vi "Parse Variant.vi"(8 "error in":errorcluster, 10 "variant":variant) -> (0 "error out":errorcluster, 1 "Types":T1[](array[typedef]), 2 "Strings":string[](array[string]), 3 "Variants":variant[](array[variant]), 4 "Types (strings)":string[](array[string]))   [LabVIEW 2020, in "Data.PG.lvclass"]
uses:
  Data.PG.lvclass
  <vilib>/Utility/Data Type/NI_Data Type.lvlib
  <vilib>/Utility/Data Type/Type Definitions/Data Type.ctl
  <vilib>/ErrorRing/Error Ring.xnode
  <vilib>/Utility/error.llb/Error Cluster From Error Code.vi
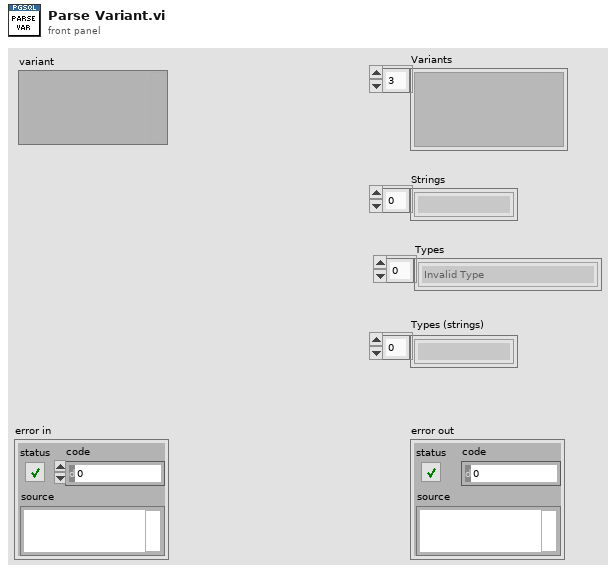
[diagram p1: front panel]
types:
  T1 = typedef "NI_Data Type.lvlib/Data Type.ctl" = enum8{"Invalid Type", "Void", "I8", "I16", "I32", "I64", "U8", "U16", "U32", "U64", "Single Float", "Double Float", "Extended Float", "Single Complex", "Double Complex", "Extended Complex", "Enum U8", "Enum U16", "Enum U32", "Enum U64", "Single Float With Unit", "Double Float With Unit", "Extended Float With Unit", "Single Complex with Unit", "Double Complex with Unit", "Extended Complex with Unit", "Boolean", "String", "Path", "Picture", "Tag", "Array", "Cluster", "Variant", "LV Variant", "Waveform", "Timestamp", "Digital Waveform", "Digital Data", "ExpressData", "Refnum", "External Data", "VI", "Poly VI", "LabVIEW Class Instance", "Fixed Point", "Set Collection", "Map Collection"}
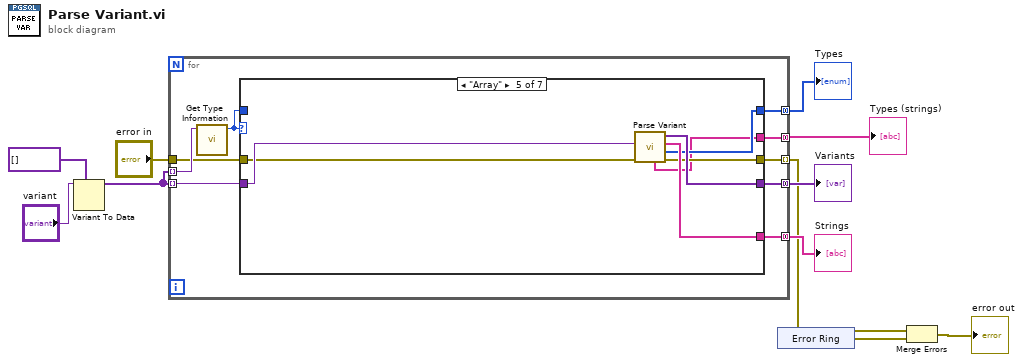
[diagram p0: block diagram]
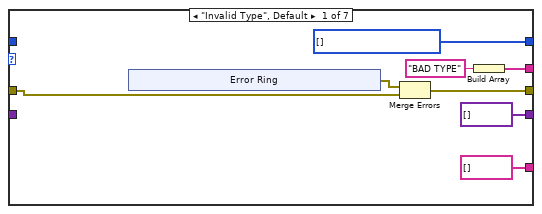
[diagram p2: hidden frame]
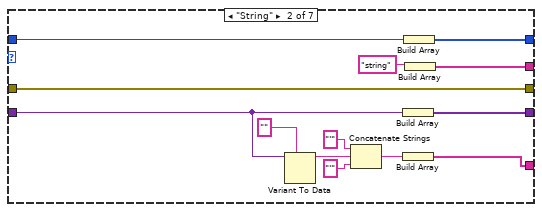
[diagram p3: hidden frame]
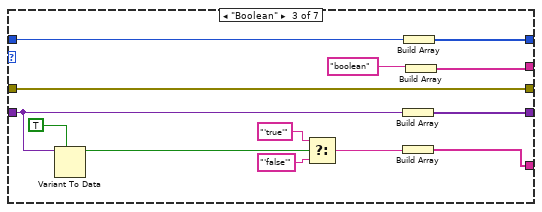
[diagram p4: hidden frame]
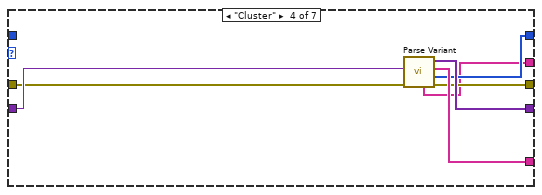
[diagram p5: hidden frame]
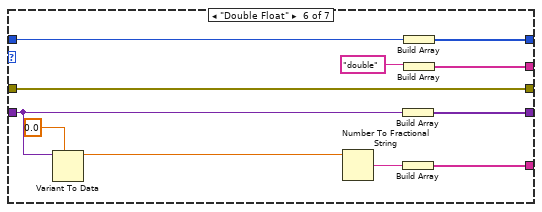
[diagram p6: hidden frame]
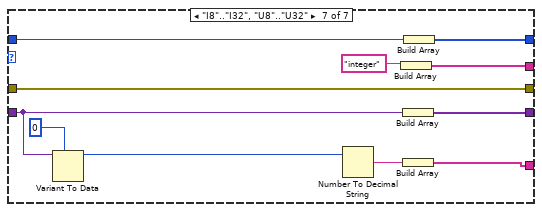
[diagram p7: hidden frame]
diagram:
  n1 = Variant To Data(type=variant[] [], Variant="variant") -> (data=w11:variant[])  [unwired: 1 in, 1 out]
  n2 = for {
    tunnel: w11 -> [w20] mode=indexing
    tunnel: w11 -> [w19] mode=indexing
    tunnel: [w17] -> w8 mode=concatenating
    tunnel: [w16] -> w7 mode=concatenating
    tunnel: [w15] -> w6 mode=concatenating
    tunnel: [w14] -> w4 mode=indexing
    tunnel: "error in" -> [w13]
    tunnel: [w12] -> w1 mode=concatenating
    n3 = call <vilib>:"Get Type Information.vi"("variant"=w20) -> ("type"=w18:T1)  [unwired: 6 in, 4 out]
    n4 = case shown="\"Array\"" w18 {
      tunnel: w19 -> [_ w38 w51 w66 w73 w77 w91]
      tunnel: [string[] [] ("Strings") w41 w54 w64 w71 w80 w89] -> w16
      tunnel: w18 -> [_ w39 w52 _ _ w82 w93]
      tunnel: [w26 w40 w53 w63 w70 w81 w92] -> w17
      tunnel: [variant[] [] ("Variants") w37 w50 w65 w72 w78 w90] -> w15
      tunnel: [w25 w36 w49 w62 w68 w76 w87] -> w14
      tunnel: w13 -> [w24 w36 w49 w61 w69 w76 w87]
      tunnel: [w22 w34 w47 w60 w67 w74 w85] -> w12
      frame "Invalid Type", Default {
        w26 = T1[] [] items=["Invalid Type", "Void", "I8", "I16", "I32", "I64", "U8", "U16", "U32", "U64", "Single Float", "Double Float", "Extended Float", "Single Complex", "Double Complex", "Extended Complex", "Enum U8", "Enum U16", "Enum U32", "Enum U64", "Single Float With Unit", "Double Float With Unit", "Extended Float With Unit", "Single Complex with Unit", "Double Complex with Unit", "Extended Complex with Unit", "Boolean", "String", "Path", "Picture", "Tag", "Array", "Cluster", "Variant", "LV Variant", "Waveform", "Timestamp", "Digital Waveform", "Digital Data", "ExpressData", "Refnum", "External Data", "VI", "Poly VI", "LabVIEW Class Instance", "Fixed Point", "Set Collection", "Map Collection"] ("Types")
        n5 = xnode "Error Ring"() -> ("error out"=w23:errorcluster)
        n6 = Merge Errors(w23, w24) -> (w25:errorcluster)
        n7 = Build Array("BAD TYPE") -> (w22:string[])
      }
      frame "String" {
        n8 = Variant To Data(type="", Variant=w38) -> (data=w45:string)  [unwired: 1 in, 1 out]
        n9 = Concatenate Strings("'" ("string"), w45, "'" ("string")) -> (w42:string)
        n10 = Build Array(w38) -> (w37:variant[])
        n11 = Build Array(w42) -> (w41:string[])
        n12 = Build Array(w39) -> (w40:T1[])
        n13 = Build Array("string") -> (w34:string[])
      }
      frame "Boolean" {
        n14 = Variant To Data(type=TRUE, Variant=w51) -> (data=w58:bool)  [unwired: 1 in, 1 out]
        n15 = Select(t="'true'", s=w58, f="'false'") -> (s? t:f=w55:string)
        n16 = Build Array(w51) -> (w50:variant[])
        n17 = Build Array(w55) -> (w54:string[])
        n18 = Build Array(w52) -> (w53:T1[])
        n19 = Build Array("boolean") -> (w47:string[])
      }
      frame "Cluster" {
        n20 = call "Parse Variant.vi"("error in"=w61, "variant"=w66) -> ("error out"=w62:errorcluster, "Types"=w63:T1[], "Strings"=w64:string[], "Variants"=w65:variant[], "Types (strings)"=w60:string[])  [unwired: 5 in]
      }
      frame "Array" {
        n21 = call "Parse Variant.vi"("error in"=w69, "variant"=w73) -> ("error out"=w68:errorcluster, "Types"=w70:T1[], "Strings"=w71:string[], "Variants"=w72:variant[], "Types (strings)"=w67:string[])  [unwired: 5 in]
      }
      frame "Double Float" {
        n22 = Variant To Data(type=0.0, Variant=w77) -> (data=w83:dbl)  [unwired: 1 in, 1 out]
        n23 = Number To Fractional String(number=w83) -> (F-format string=w79:string)  [unwired: 3 in]
        n24 = Build Array(w77) -> (w78:variant[])
        n25 = Build Array(w79) -> (w80:string[])
        n26 = Build Array(w82) -> (w81:T1[])
        n27 = Build Array("double") -> (w74:string[])
      }
      frame "I8".."I32", "U8".."U32" {
        n28 = Variant To Data(type=0, Variant=w91) -> (data=w94:i32)  [unwired: 1 in, 1 out]
        n29 = Number To Decimal String(number=w94) -> (decimal integer string=w88:string)  [unwired: 1 in]
        n30 = Build Array("integer") -> (w85:string[])
        n31 = Build Array(w91) -> (w90:variant[])
        n32 = Build Array(w88) -> (w89:string[])
        n33 = Build Array(w93) -> (w92:T1[])
      }
    }
  }
  "Variants" <- w6
  "Types" <- w8
  "Strings" <- w7
  "Types (strings)" <- w1
  n34 = xnode "Error Ring"() -> ("error out"=w2:errorcluster)
  n35 = Merge Errors(w4, w2) -> (→"error out":errorcluster)
